vi "DSF.Engine.Plugin.Initialize.vi"(8 "error in (no error)":errorcluster, 9 "Transceiver":refnum<class "Transceiver.lvclass">, 10 "Transfer Groups":refnum<class "DSF.Engine.Transfer Group.lvclass">[](array[class]), 11 "Plugin in":refnum<class "DSF.Engine.Plugin.lvclass">) -> (0 "error out":errorcluster, 3 "Plugin out":refnum<class "DSF.Engine.Plugin.lvclass">)   [LabVIEW 2017, in "Data Sharing Framework Engine.lvlib" / "DSF.Engine.Plugin.lvclass"]
uses:
  DSF.Engine.Plugin.lvclass
  Transfer/DSF.Engine.Transfer Group.lvclass
  Source/Data Sharing Framework Core/Engine/Transceiver/Transceiver/Transceiver.lvclass
  DSF.Engine.Plugin.lvclass/DSF.Engine.Plugin.ctl
  Source/Data Sharing Framework Core/Engine/Timing/Engine Timing.lvclass/Engine Timing.ctl
  Source/Data Sharing Framework Core/Engine/Debug/Debug Flags/Debug Flags.lvclass/Debug Flags.ctl
  Source/Data Sharing Framework Core/Engine/Execution/Pool/Pool/Pool.lvclass/Pool.ctl
  Source/Data Sharing Framework Core/Engine/Debug/Debug Flags FIFO/Debug Flags FIFO.lvclass/Debug Flags FIFO.ctl
  Source/Data Sharing Framework Core/Engine/Execution/Pool/Pool/Read FIFO.vi
  Source/Data Sharing Framework Core/Engine/Execution/Pool/Pool/Write FIFO.vi
  Source/Data Sharing Framework Core/Engine/Execution/Pool/Pool/Get FIFO.vi
  Source/Data Sharing Framework Core/Engine/Execution/Pool/Pool/Get Debug Flags.vi
  Source/Data Sharing Framework Core/Engine/Debug/Debug Flags FIFO/Get Infinite Timeouts.vi
  Source/Data Sharing Framework Core/Engine/Execution/Pool/Pool ID/Pool ID.lvclass
  C:/github/data-sharing-framework/Source/Data Sharing Framework Core/Engine/Execution/Pool/Pool/Pool.lvclass
  Source/Data Sharing Framework Core/Engine/Transceiver/Transceiver Thread/Transceiver Thread.lvclass
  Thread Parameters/Thread Parameters.lvclass
  Source/Data Sharing Framework Core/Engine/Timing/Engine Timing.lvclass
  Source/Data Sharing Framework Core/Engine/Debug/Debug Flags/Debug Flags.lvclass
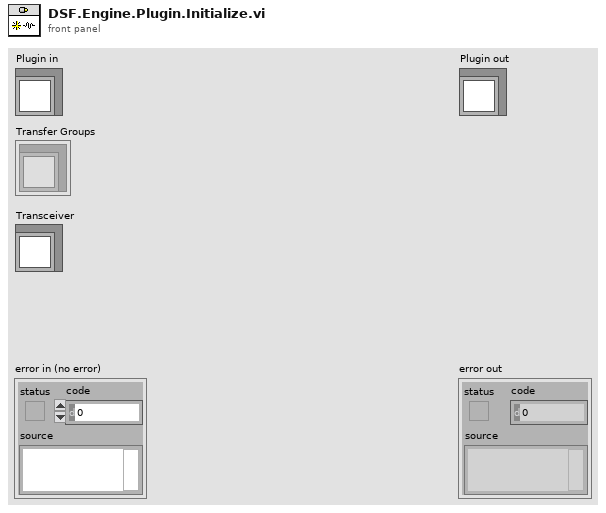
[diagram p1: front panel]
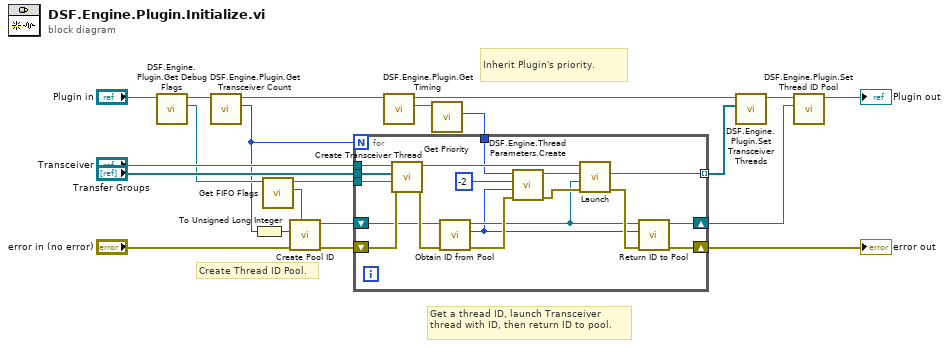
[diagram p0: block diagram]
diagram:
  # "Inherit Plugin's priority."
  # "Get a thread ID, launch Transceiver thread with ID, then return ID to pool."
  # "Create Thread ID Pool."
  n1 = call "DSF.Engine.Plugin.Get Debug Flags.vi"("Plugin in"="Plugin in") -> ("Debug Flags"=w2:refnum<class "Debug Flags.lvclass">, "Plugin out"=w9:refnum<class "DSF.Engine.Plugin.lvclass">)  [unwired: 9 in]
  n2 = call "DSF.Engine.Plugin.Get Transceiver Count.vi"("Plugin in"=w9) -> ("transceiver count"=w1:i32, "Plugin out"=w21:refnum<class "DSF.Engine.Plugin.lvclass">)  [unwired: 9 in]
  n3 = To Unsigned Long Integer(number=w1) -> (unsigned 32bit integer=w15:u32)
  n4 = call "Get FIFO Flags.vi"("Debug Flags in"=w2) -> ("FIFO"=w8:refnum<class "Debug Flags FIFO.lvclass">, "Debug Flags out"=w7:refnum<class "Debug Flags.lvclass">)  [unwired: 9 in]
  n5 = call "Create Pool ID.vi"("FIFO Debug Flags"=w8, "error in (no error)"="error in (no error)", "number of IDs"=w15) -> ("error out"=w6:errorcluster, "ID Pool out"=w16:refnum<class "Pool ID.lvclass">)  [unwired: 7 in]
  n6 = call "DSF.Engine.Plugin.Get Timing.vi"("Plugin in"=w21) -> ("Timing"=w18:refnum<class "Engine Timing.lvclass">, "Plugin out"=w14:refnum<class "DSF.Engine.Plugin.lvclass">)  [unwired: 9 in]
  n7 = call "Get Priority.vi"("Timing in"=w18) -> ("Priority"=w17:u64)  [unwired: 9 in, 1 out]
  n8 = for {
    N: w1 -> [_]
    tunnel: "Transceiver" -> [w39]
    shift-right: [w28] -> w20
    shift-left: w6 -> [w38]
    tunnel: w17 -> [w25]
    tunnel: [w29] -> w13 mode=indexing
    shift-right: [w24] -> w10
    shift-left: w16 -> [w26]
    tunnel: w7 -> [w23]
    tunnel: "Transfer Groups" -> [w22]
    n9 = call "Create Transceiver Thread.vi"("error in (no error)"=w38, "Debug Flags"=w23, "Transfer Groups"=w22, "Transceiver type"=w39) -> ("error out"=w27:errorcluster, "Transceiver Thread out"=w30:refnum<class "Transceiver Thread.lvclass">)  [unwired: 6 in]
    n10 = call "Obtain ID from Pool.vi"("error in (no error)"=w27, "ID Pool in"=w26) -> ("error out"=w36:errorcluster, "id"=w31:i32, "ID Pool out"=w33:refnum<class "Pool ID.lvclass">)  [unwired: 6 in, 1 out]
    n11 = call "DSF.Engine.Thread Parameters.Create.vi"("error in (no error)"=w36, "id"=w31, "processor"=-2, "priority"=w25) -> ("error out"=w35:errorcluster, "Thread Parameters"=w32:refnum<class "Thread Parameters.lvclass">)  [unwired: 6 in]
    n12 = call "Launch.vi"("error in (no error)"=w35, "Thread ID Pool"=w33, "Thread Parameters"=w32, "Transceiver Thread in"=w30) -> ("error out"=w34:errorcluster, "Interface"=w29:refnum<class "Transceiver Interface.lvclass">)  [unwired: 5 in, 1 out]
    n13 = call "Return ID to Pool.vi"("error in (no error)"=w34, "id"=w31, "ID Pool in"=w33) -> ("error out"=w28:errorcluster, "ID Pool out"=w24:refnum<class "Pool ID.lvclass">)  [unwired: 6 in, 1 out]
  }
  "error out" <- w20
  n14 = call "DSF.Engine.Plugin.Set Transceiver Threads.vi"("Transceiver Threads"=w13, "Plugin in"=w14) -> ("Plugin out"=w12:refnum<class "DSF.Engine.Plugin.lvclass">)  [unwired: 9 in]
  n15 = call "DSF.Engine.Plugin.Set Thread ID Pool.vi"("Thread ID Pool"=w10, "Plugin in"=w12) -> ("Plugin out"=→"Plugin out":refnum<class "DSF.Engine.Plugin.lvclass">)  [unwired: 9 in]
